vi "Pressure_Control.vi"() -> ()   [LabVIEW 2019]
uses:
  Pressure Control SubVIs/Device Data.ctl
  DevHandshake_elt.ctl
  <vilib>/Platform/TimedLoop/XDataNode/timing_clust.ctl
  <vilib>/Platform/TimedLoop/XDataNode/nitl_modes.ctl
  <vilib>/Platform/TimedLoop/XDataNode/wakeup.ctl
  octo-master/octo-master/DevHandshake.ctl
  <vilib>/platform/TimedLoop/XDataNode/XDataNode.xnode
  <vilib>/Platform/TimedLoop/XDataNode/XDNodeRunTimeDep.lvlib
panel:
  out "DevSave":T1
  out "Error Out":errorcluster
  in  "Current pressure status":string
  in  "Pressure tolerance %":sgl
  out "Status":string="NOT SYNC'D"
  out "Dev ID":string="pressureControl"
  in  "DevNum":i16=5
  out "Warning":bool
  out "Device Data":T2={"COM"=4, "Baud"=19200, "IDH"=0, "IDM"=0, "IDL"=0, "IDS"=0} {"IDS" format="%.0x"; "IDL" format="%.0x"; "IDM" format="%.0x"; "IDH" format="%.0x"}
  in  "SetPoint":sgl format="%.2f"
  in  "Write setpoint":bool
  in  "Read current setpoint":bool
  out "Unit":string
  out "Set Point Value":sgl format="%.2f"
  out "SetPoint %":sgl format="%.2f"
  in  "Lock to Network":bool
  out "Pressure Unit":string
  out "Pressure":sgl format="%.2f"
  in  "Read current pressure":bool
  in  "Message":string
  out "Function Output Comment":string
  in  "Start device":bool
  in  "Stop Button":bool
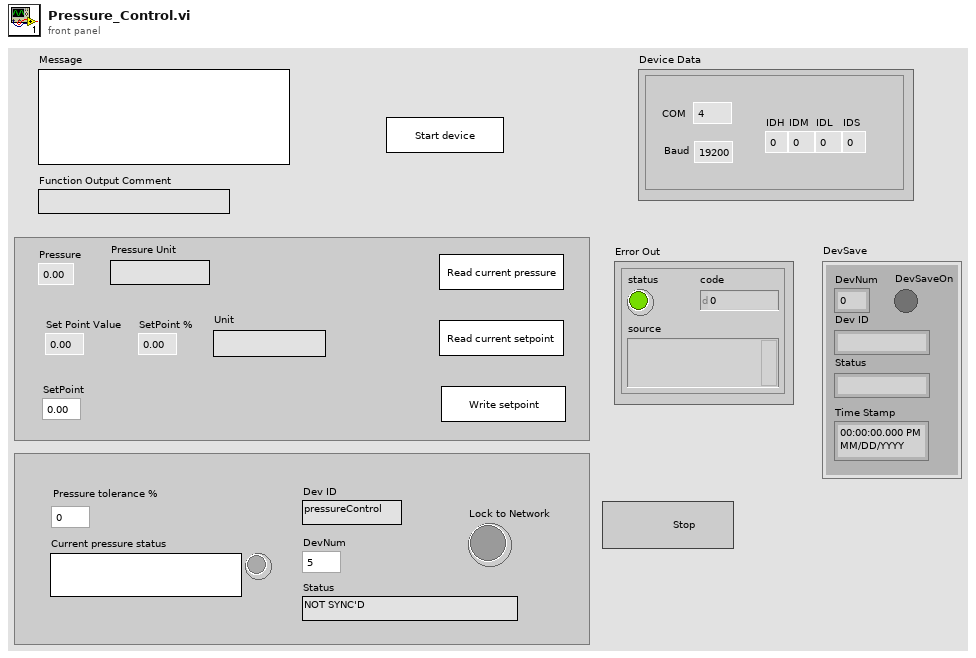
[diagram p1: front panel]
types:
  T1 = typedef "DevHandshake_elt.ctl" = cluster{"DevSaveOn":bool, "DevNum":i16, "Dev ID":string, "Status":string, "Time Stamp":timestamp}
  T2 = typedef "Device Data.ctl" = cluster{"COM":i32, "Baud":i32, "IDH":u8, "IDM":u8, "IDL":u8, "IDS":u8}
  T3 = typedef "XDNodeRunTimeDep.lvlib/timing_clust.ctl" = cluster{"Expected End [f-1]":u64, "Actual End [f-1]":u64, "Finished Late? [f-1]":bool, "Expected End [i-1]":u64, "Actual End [i-1]":u64, "Finished Late? [i-1]":bool, "Expected Start [i]":u64, "Actual Start [i]":u64, "Expected Start [f]":u64, "Actual Start [f]":u64, "Source Name":string, "Structure Name":string, "Period":i64, "Deadline":i64, "Offset":i64, "Start":i64, "Priority":i32, "Timeout":i32, "Mode":T4, "Wakeup Reason":T5, "Error":errorcluster, "Source Type":string, "Secondary Source Type":string, "Global End Time":u64, "Global Start Time":u64, "Frame Duration":u64, "Iteration Duration":u64, "Assigned CPU":i32, "I/O Scan Engine Mode":u32}
  T4 = typedef "XDNodeRunTimeDep.lvlib/nitl_modes.ctl" = enum32{"No Change", "Process missed periods, maintain original phase", "Discard missed periods, maintain original phase", "Process missed periods, ignore original phase", "Discard missed periods, ignore original phase"}
  T5 = typedef "XDNodeRunTimeDep.lvlib/wakeup.ctl" = enum32{"Normal", "Aborted", "Asynchronous wakeup", "Timing source error", "Timed loop error", "Timeout"}
  T6 = typedef "DevHandshake.ctl" = cluster{"DevSaveOn":bool, "DevNum":i16, "Dev ID":string, "Status":string, "Time Stamp":timestamp}[]
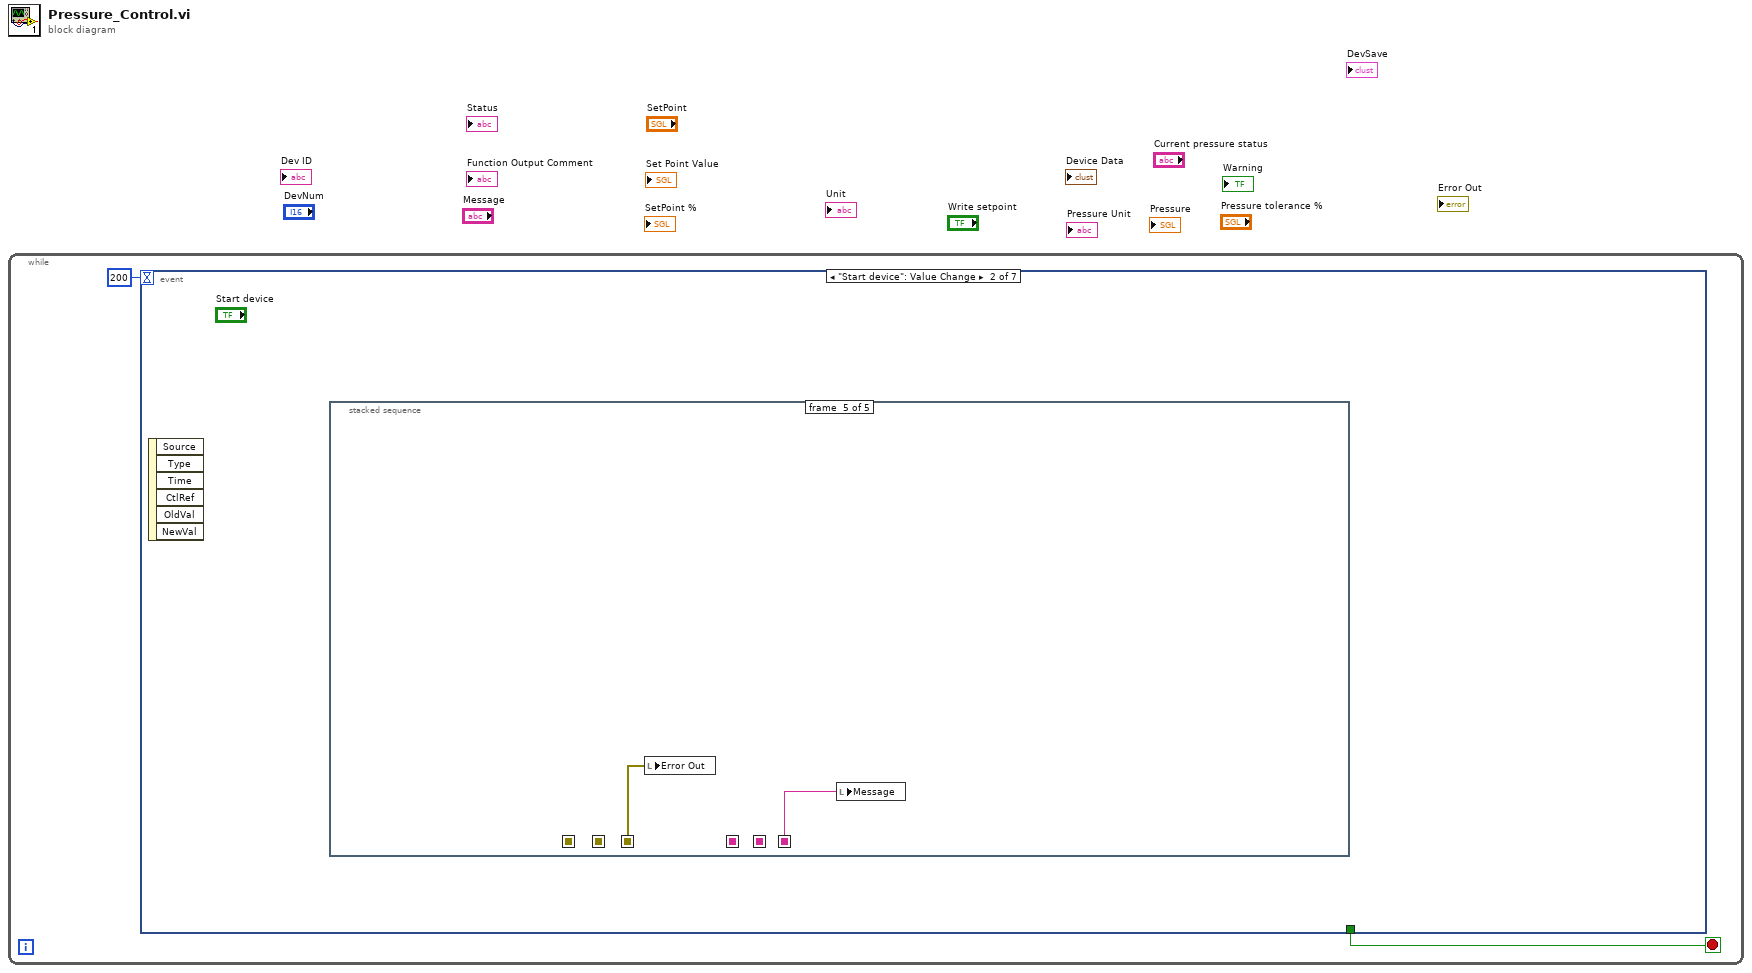
[diagram p0: block diagram]
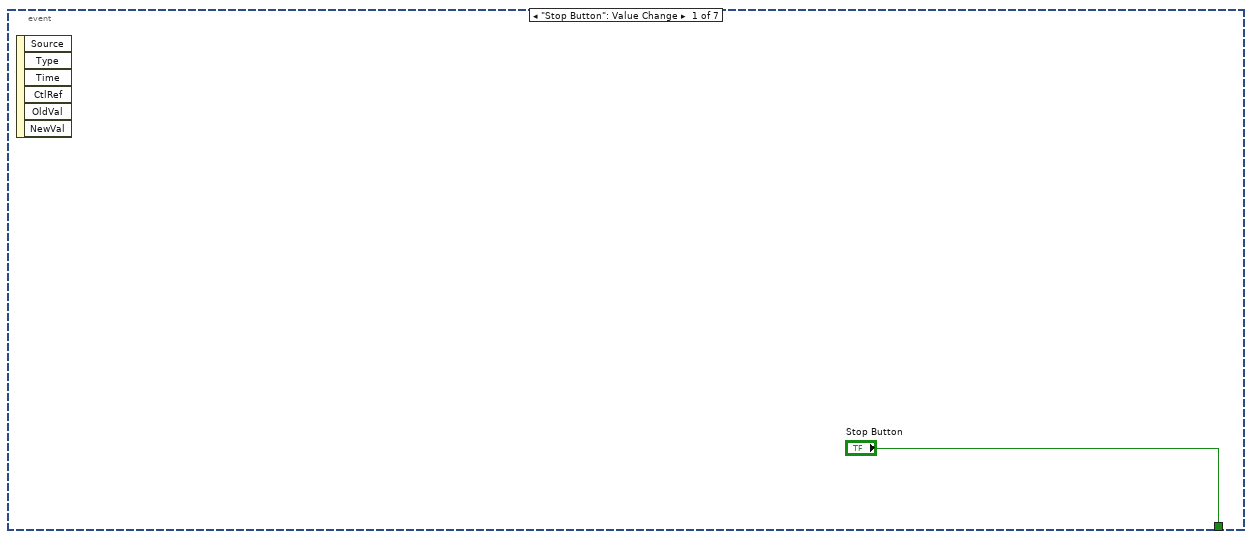
[diagram p2: hidden frame]
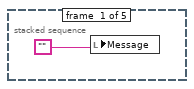
[diagram p3: hidden frame]
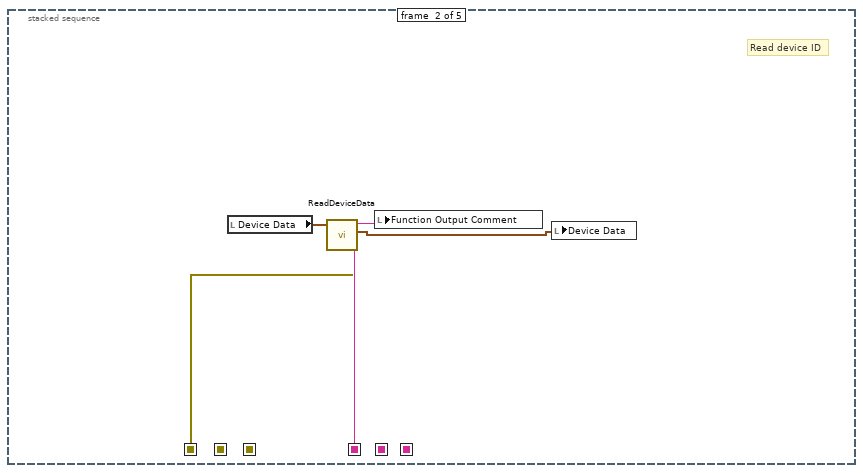
[diagram p4: hidden frame]
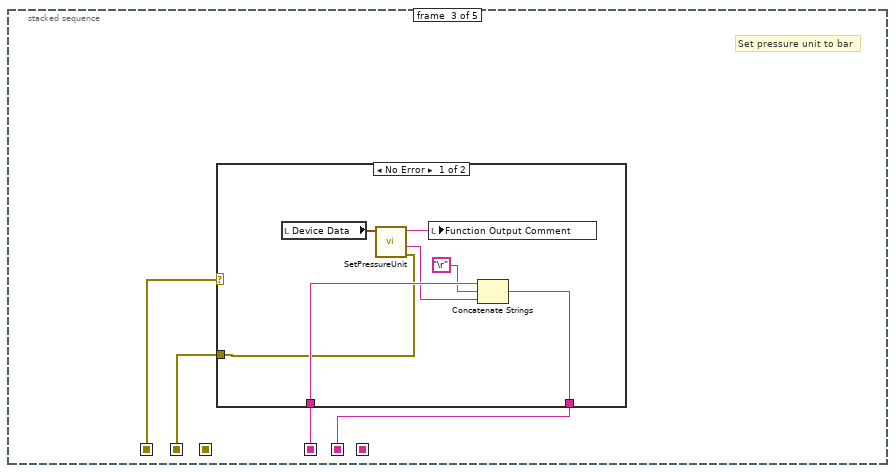
[diagram p5: hidden frame]
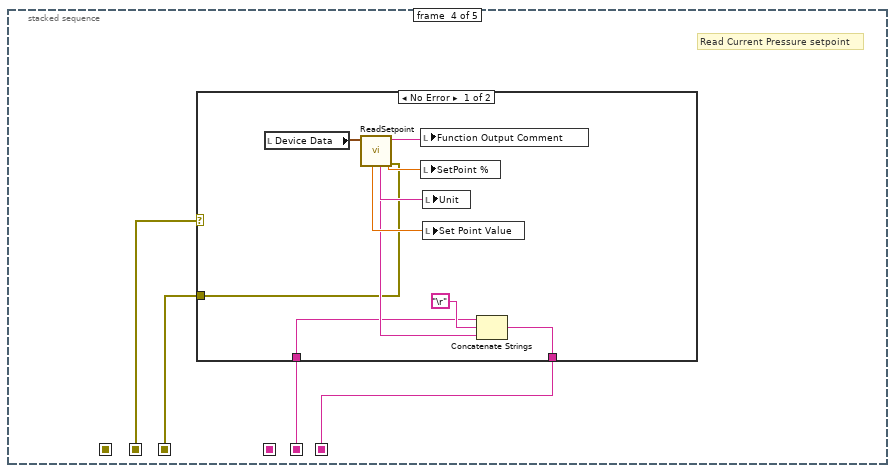
[diagram p7: hidden frame]
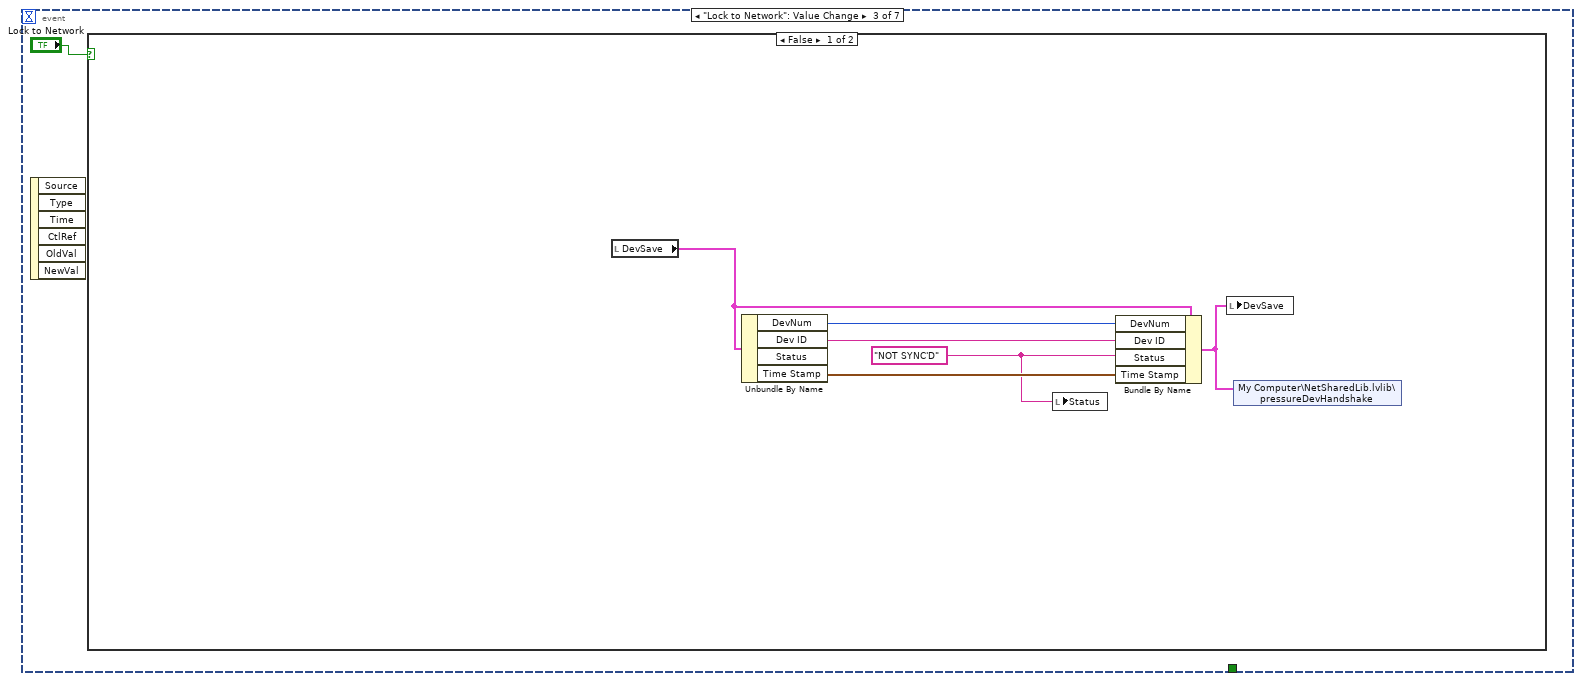
[diagram p9: hidden frame]
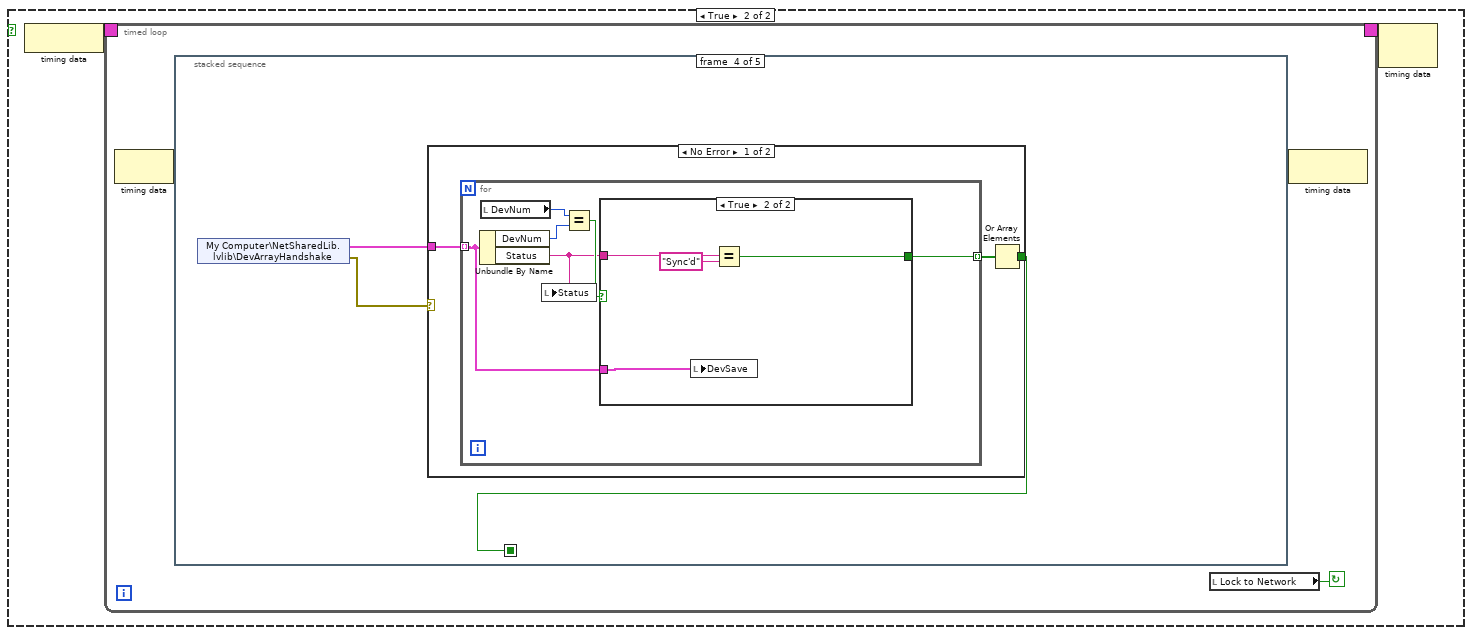
[diagram p10: hidden frame]
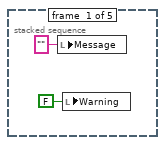
[diagram p11: hidden frame]
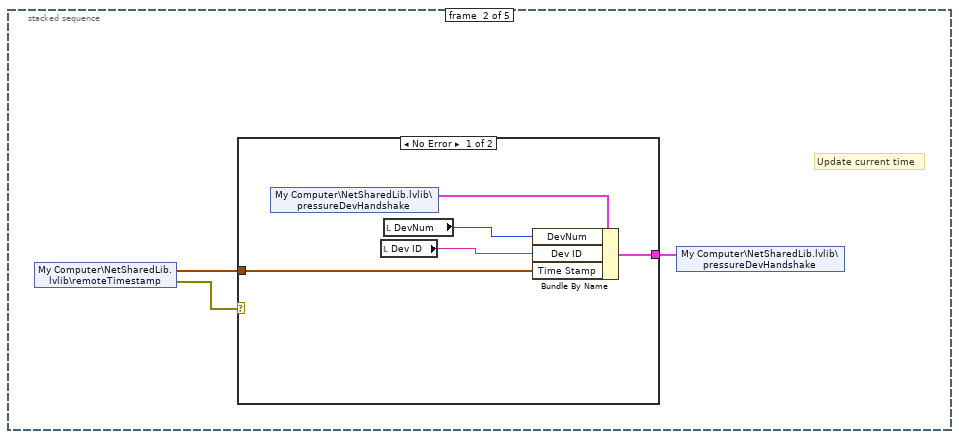
[diagram p12: hidden frame]
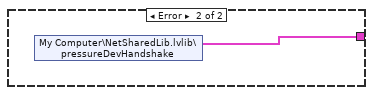
[diagram p13: hidden frame]
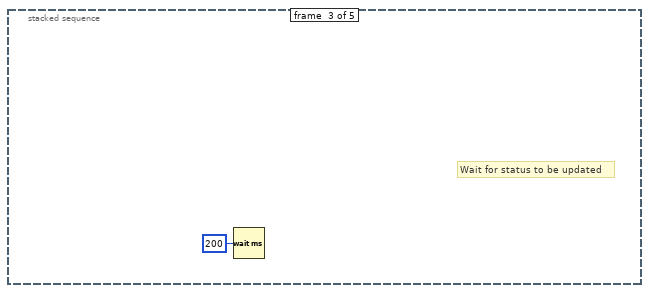
[diagram p14: hidden frame]
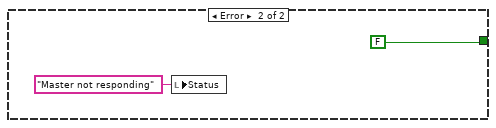
[diagram p16: hidden frame]
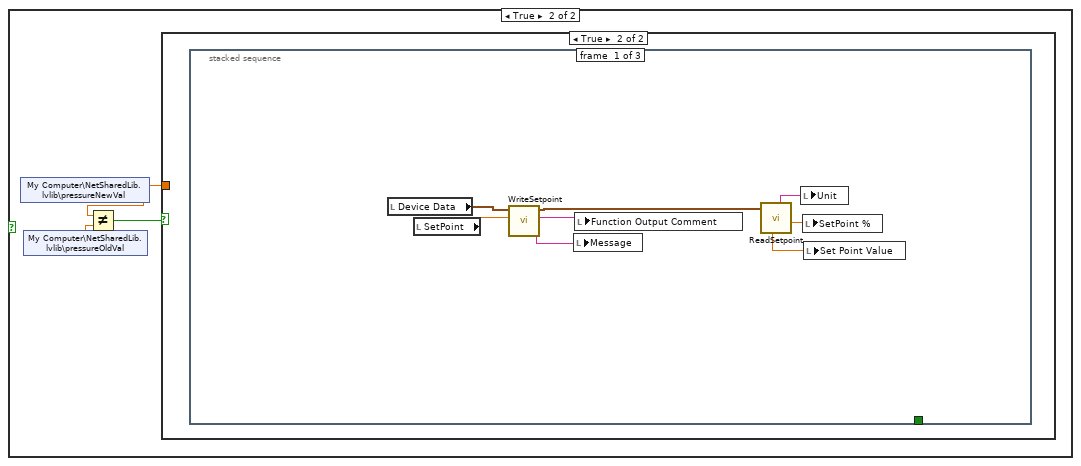
[diagram p18: hidden frame]
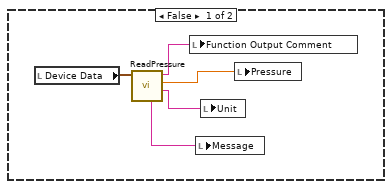
[diagram p19: hidden frame]
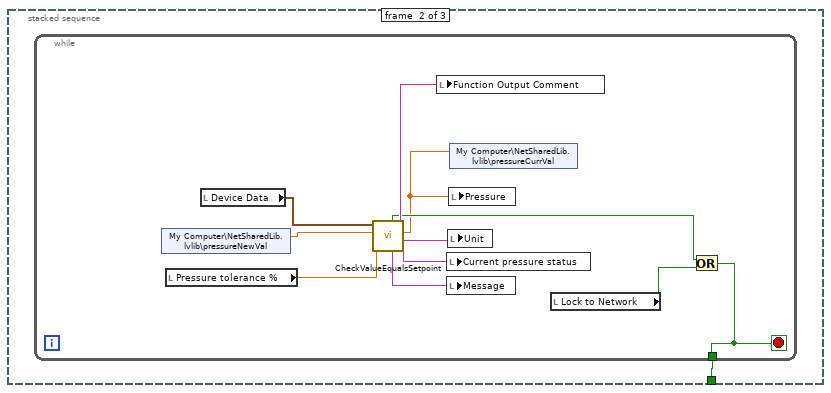
[diagram p20: hidden frame]
diagram:
  n1 = while {
    stop <- w2 stop-if-true
    n2 = event shown="[1] \"Start device\": Value Change" {
      selector: _ -> [_ _ _ _ _ _ _]
      dyn-events: _ -> [_ _ _ _ _ _ _]
      timeout: 200 -> [_ _ _ _ _ _ _]
      tunnel: ["Stop Button" _ _ _ _ _ _] -> w2
      event "Stop Button": Value Change {
        n3 = event-data() -> ()  [unwired: 1 in, 6 out]
      }
      event "Start device": Value Change {
        n4 = event-data() -> ()  [unwired: 1 in, 6 out]
        n5 = stacked-sequence {
          seq-local: [_ w8 _ _ _] -> [_ _ w13 _ _]
          seq-local: [_ _ w12 _ _] -> [_ _ _ w26 _]
          seq-local: [_ _ _ w25 _] -> [_ _ _ _ w40]
          seq-local: [_ w5 _ _ _] -> [_ _ w11 _ _]
          seq-local: [_ _ w10 _ _] -> [_ _ _ w24 _]
          seq-local: [_ _ _ w23 _] -> [_ _ _ _ w39]
          frame #0 {
            n6 = local write "Message"("") -> ()
          }
          frame #1 {
            # "Read device ID"
            n7 = local read "Device Data"() -> (w6:T2)
            n8 = call "ReadDeviceData.vi"("Device Data in"=w6) -> ("Error Out"=w5:errorcluster, "Message"=w8:string, "Device Data out"=w7:T2, "Function Output Comment"=w9:string)  [unwired: 7 in]
            n9 = local write "Function Output Comment"(w9) -> ()
            n10 = local write "Device Data"(w7) -> ()
          }
          frame #2 {
            # "Set pressure unit to bar"
            n11 = case shown="No Error" w11 {
              selector: w11 -> [_ w21]
              tunnel: w13 -> [w18 w22]
              tunnel: [w15 w22] -> w12
              tunnel: [w14 w21] -> w10
              frame No Error {
                n12 = local read "Device Data"() -> (w19:T2)
                n13 = call "SetPressureUnit.vi"("Device Data in"=w19) -> ("Error Out"=w14:errorcluster, "Message"=w17:string, "Function Output Comment"=w20:string)  [unwired: 7 in, 1 out]
                n14 = local write "Function Output Comment"(w20) -> ()
                n15 = Concatenate Strings(w18, "\r", w17) -> (w15:string)
              }
              frame Error {
              }
            }
          }
          frame #3 {
            # "Read Current Pressure setpoint"
            n16 = case shown="No Error" w24 {
              selector: w24 -> [_ w38]
              tunnel: w26 -> [w29 w37]
              tunnel: [w28 w37] -> w25
              tunnel: [w27 w38] -> w23
              frame No Error {
                n17 = local read "Device Data"() -> (w32:T2)
                n18 = call "ReadSetpoint.vi"("Device Data in"=w32) -> ("Error Out"=w27:errorcluster, "SetPoint %"=w35:sgl, "Function Output Comment"=w36:string, "Unit"=w33:string, "Message"=w30:string, "SetPointValue"=w34:sgl)  [unwired: 4 in, 1 out]
                n19 = local write "Function Output Comment"(w36) -> ()
                n20 = local write "SetPoint %"(w35) -> ()
                n21 = local write "Unit"(w33) -> ()
                n22 = local write "Set Point Value"(w34) -> ()
                n23 = Concatenate Strings(w29, "\r", w30) -> (w28:string)
              }
              frame Error {
              }
            }
          }
          frame #4 {
            n24 = local write "Error Out"(w39) -> ()
            n25 = local write "Message"(w40) -> ()
          }
        }
      }
      event "Lock to Network": Value Change {
        n26 = event-data() -> ()  [unwired: 1 in, 6 out]
        n27 = case shown="False" "Lock to Network" {
          frame False {
            w42 = "NOT SYNC'D"
            n28 = local read "DevSave"() -> (w43:T1)
            n29 = Unbundle By Name(w43) -> ("DevNum"=w47:i16, "Dev ID"=w46:string, "Time Stamp"=w45:timestamp)  [unwired: 1 out]
            n30 = local write "Status"(w42) -> ()
            n31 = Bundle By Name(cluster=w43, "DevNum"=w47, "Dev ID"=w46, "Status"=w42, "Time Stamp"=w45) -> (w44:T1)
            n32 = local write "DevSave"(w44) -> ()
            n33 = shared-variable "My Computer\\NetSharedLib.lvlib\\pressureDevHandshake"(w44) -> ()  [unwired: 1 in, 1 out]
          }
          frame True {
            n34 = node-c288() -> (w49:T3)
            n35 = timed-loop {
              timing: w49 -> [_]
              timing-out: [_] -> w48
              stop <- w50 continue-if-true
              n36 = node-c288() -> ()  [unwired: 1 in, 1 out]
              n37 = stacked-sequence {
                seq-local: [_ _ _ w66 _] -> [_ _ _ _ w84]
                frame #0 {
                  n38 = local write "Message"("" ("Message")) -> ()
                  n39 = local write "Warning"(FALSE ("Warning")) -> ()
                }
                frame #1 {
                  # "Update current time"
                  n40 = shared-variable "My Computer\\NetSharedLib.lvlib\\remoteTimestamp"() -> (w57:timestamp, error out=w55:errorcluster)  [unwired: 1 in]
                  n41 = case shown="No Error" w55 {
                    tunnel: w57 -> [w60 _]
                    tunnel: [w58 w63] -> w56
                    frame No Error {
                      n42 = shared-variable "My Computer\\NetSharedLib.lvlib\\pressureDevHandshake"() -> (w59:T1)  [unwired: 1 in, 1 out]
                      n43 = local read "Dev ID"() -> (w62:string)
                      n44 = local read "DevNum"() -> (w61:i16)
                      n45 = Bundle By Name(cluster=w59, "DevNum"=w61, "Dev ID"=w62, "Time Stamp"=w60) -> (w58:T1)
                    }
                    frame Error {
                      n46 = shared-variable "My Computer\\NetSharedLib.lvlib\\pressureDevHandshake"() -> (w63:T1)  [unwired: 1 in, 1 out]
                    }
                  }
                  n47 = shared-variable "My Computer\\NetSharedLib.lvlib\\pressureDevHandshake"(w56) -> ()  [unwired: 1 in, 1 out]
                }
                frame #2 {
                  # "Wait for status to be updated"
                  n48 = Wait (ms)(milliseconds to wait=u32 200) -> ()  [unwired: 1 out]
                }
                frame #3 {
                  n49 = shared-variable "My Computer\\NetSharedLib.lvlib\\DevArrayHandshake"() -> (w67:T6, error out=w65:errorcluster)  [unwired: 1 in]
                  n50 = case shown="No Error" w65 {
                    tunnel: w67 -> [w70 _]
                    tunnel: [w68 FALSE] -> w66
                    frame No Error {
                      n51 = for {
                        tunnel: w70 -> [w71] mode=indexing
                        tunnel: [w73] -> w69 mode=indexing
                        n52 = Unbundle By Name(w71) -> ("DevNum"=w76:i16, "Status"=w72:string)
                        n53 = local read "DevNum"() -> (w75:i16)
                        n54 = local write "Status"(w72) -> ()
                        n55 = Equal?(x=w75, y=w76) -> (x = y?=w74:bool)
                        n56 = case shown="True" w74 {
                          selector: w74 -> [w77 _]
                          tunnel: w72 -> [_ w81]
                          tunnel: [w77 w79] -> w73
                          tunnel: w71 -> [_ w78]
                          frame False {
                          }
                          frame True {
                            n57 = local write "DevSave"(w78) -> ()
                            n58 = Equal?(x=w81, y="Sync'd") -> (x = y?=w79:bool)
                          }
                        }
                      }
                      n59 = Or Array Elements(Boolean array=w69) -> (logical OR=w68:bool)
                    }
                    frame Error {
                      n60 = local write "Status"("Master not responding" ("Status")) -> ()
                    }
                  }
                }
                frame #4 {
                  n61 = case shown="False" w84 {
                    frame False {
                    }
                    frame True {
                      n62 = shared-variable "My Computer\\NetSharedLib.lvlib\\pressureNewVal"() -> (w85:sgl)  [unwired: 1 in, 1 out]
                      n63 = shared-variable "My Computer\\NetSharedLib.lvlib\\pressureOldVal"() -> (w87:sgl)  [unwired: 1 in, 1 out]
                      n64 = Not Equal?(x=w85, y=w87) -> (x != y?=w86:bool)
                      n65 = case shown="True" w86 {
                        tunnel: w85 -> [_ _]
                        frame False {
                          n66 = local read "Device Data"() -> (w92:T2)
                          n67 = call "ReadPressure.vi"("Device Data"=w92) -> ("Unit"=w88:string, "Pressure"=w90:sgl, "Function Output Comment"=w91:string, "Message"=w89:string)  [unwired: 7 in]
                          n68 = local write "Function Output Comment"(w91) -> ()
                          n69 = local write "Message"(w89) -> ()
                          n70 = local write "Unit"(w88) -> ()
                          n71 = local write "Pressure"(w90) -> ()
                        }
                        frame True {
                          n72 = stacked-sequence {
                            tunnel: [_ w101 _] -> _
                            frame #0 {
                              n73 = local read "Device Data"() -> (w96:T2)
                              n74 = local read "SetPoint"() -> (w98:sgl)
                              n75 = call "WriteSetpoint.vi"("SetPoint"=w98, "Device Data"=w96) -> ("Message"=w97:string, "Function Output Comment"=w99:string, "Device Data OUT"=w100:T2)  [unwired: 6 in]
                              n76 = local write "Message"(w97) -> ()
                              n77 = local write "Function Output Comment"(w99) -> ()
                              n78 = call "ReadSetpoint.vi"("Device Data in"=w100) -> ("SetPoint %"=w95:sgl, "Unit"=w93:string, "SetPointValue"=w94:sgl)  [unwired: 4 in, 4 out]
                              n79 = local write "Unit"(w93) -> ()
                              n80 = local write "SetPoint %"(w95) -> ()
                              n81 = local write "Set Point Value"(w94) -> ()
                            }
                            frame #1 {
                              n82 = while {
                                tunnel: [w104] -> w101
                                stop <- w104 stop-if-true
                                n83 = shared-variable "My Computer\\NetSharedLib.lvlib\\pressureNewVal"() -> (w107:sgl)  [unwired: 1 in, 1 out]
                                n84 = local read "Pressure tolerance %"() -> (w108:sgl)
                                n85 = local read "Device Data"() -> (w112:T2)
                                n86 = call "CheckValueEqualsSetpoint.vi"("Pressure tolerance %"=w108, "PressureNewVal"=w107, "Device Data"=w112) -> ("Current pressure status"=w106:string, "Unit"=w109:string, "Pressure"=w102:sgl, "Function Output Comment"=w111:string, "Message"=w110:string, "PeqPSet ?"=w105:bool)  [unwired: 3 in]
                                n87 = local write "Function Output Comment"(w111) -> ()
                                n88 = local write "Current pressure status"(w106) -> ()
                                n89 = local write "Message"(w110) -> ()
                                n90 = local write "Unit"(w109) -> ()
                                n91 = local write "Pressure"(w102) -> ()
                                n92 = shared-variable "My Computer\\NetSharedLib.lvlib\\pressureCurrVal"(w102) -> ()  [unwired: 1 in, 1 out]
                                n93 = local read "Lock to Network"() -> (w103:bool)
                                n94 = Or(x=w105, y=w103) -> (x .or. y?=w104:bool)
                              }
                            }
                            frame #2 {
                              n95 = local read "Lock to Network"() -> (w113:bool)
                              n96 = case shown="True" w113 {
                                frame False {
                                n97 = local read "Current pressure status"() -> (w117:string)
                                n98 = Concatenate Strings(w117, "\r" ("string"), "Connection to network was unlocked by user  " ("string")) -> (w114:string)
                                n99 = local write "Current pressure status"(w114) -> ()
                                }
                                frame True {
                                n100 = shared-variable "My Computer\\NetSharedLib.lvlib\\pressureNewVal"() -> (w118:sgl)  [unwired: 1 in, 1 out]
                                n101 = shared-variable "My Computer\\NetSharedLib.lvlib\\pressureOldVal"(w118) -> ()  [unwired: 1 in, 1 out]
                                }
                              }
                            }
                          }
                        }
                      }
                    }
                  }
                }
              }
              n102 = local read "Lock to Network"() -> (w50:bool)
              n103 = node-c288() -> ()  [unwired: 1 in, 1 out]
            }
            n104 = node-c288(w48) -> ()  [unwired: 1 out]
          }
        }
      }
      event "Read current pressure": Value Change {
        n105 = event-data() -> ()  [unwired: 1 in, 6 out]
        n106 = local read "Device Data"() -> (w122:T2)
        n107 = call "ReadPressure.vi"("Device Data"=w122) -> ("Unit"=w123:string, "Pressure"=w121:sgl, "Function Output Comment"=w125:string, "Message"=w124:string)  [unwired: 7 in]
        n108 = local write "Pressure Unit"(w123) -> ()
        n109 = local write "Message"(w124) -> ()
        n110 = local write "Function Output Comment"(w125) -> ()
        n111 = shared-variable "My Computer\\NetSharedLib.lvlib\\pressureCurrVal"(w121) -> ()  [unwired: 1 in, 1 out]
        n112 = local write "Pressure"(w121) -> ()
      }
      event "Read current setpoint": Value Change {
        n113 = event-data() -> ()  [unwired: 1 in, 6 out]
        n114 = local read "Device Data"() -> (w131:T2)
        n115 = call "ReadSetpoint.vi"("Device Data in"=w131) -> ("SetPoint %"=w129:sgl, "Function Output Comment"=w126:string, "Unit"=w130:string, "Message"=w127:string, "SetPointValue"=w128:sgl)  [unwired: 4 in, 2 out]
        n116 = local write "Message"(w127) -> ()
        n117 = local write "Unit"(w130) -> ()
        n118 = local write "Set Point Value"(w128) -> ()
        n119 = local write "Function Output Comment"(w126) -> ()
        n120 = local write "SetPoint %"(w129) -> ()
      }
      event "Write setpoint": Value Change {
        n121 = event-data() -> ()  [unwired: 1 in, 6 out]
        n122 = stacked-sequence {
          frame #0 {
            n123 = local read "Device Data"() -> (w132:T2)
            n124 = local read "SetPoint"() -> (w134:sgl)
            n125 = call "WriteSetpoint.vi"("SetPoint"=w134, "Device Data"=w132) -> ("Message"=w133:string, "Function Output Comment"=w135:string)  [unwired: 6 in, 1 out]
            n126 = local write "Function Output Comment"(w135) -> ()
            n127 = local write "Message"(w133) -> ()
          }
          frame #1 {
            n128 = local read "Device Data"() -> (w141:T2)
            n129 = call "ReadSetpoint.vi"("Device Data in"=w141) -> ("SetPoint %"=w140:sgl, "Function Output Comment"=w136:string, "Unit"=w138:string, "Message"=w137:string, "SetPointValue"=w139:sgl)  [unwired: 4 in, 2 out]
            n130 = local write "SetPoint %"(w140) -> ()
            n131 = local write "Set Point Value"(w139) -> ()
            n132 = local write "Function Output Comment"(w136) -> ()
            n133 = local write "Message"(w137) -> ()
            n134 = local write "Unit"(w138) -> ()
          }
        }
      }
      event Timeout {
        n135 = event-data() -> ()  [unwired: 1 in, 3 out]
        n136 = local read "Device Data"() -> (w143:T2)
        n137 = call "ReadPressure.vi"("Device Data"=w143) -> ("Unit"=w144:string, "Pressure"=w142:sgl, "Function Output Comment"=w146:string, "Message"=w145:string)  [unwired: 7 in]
        n138 = local write "Function Output Comment"(w146) -> ()
        n139 = local write "Pressure Unit"(w144) -> ()
        n140 = local write "Message"(w145) -> ()
        n141 = shared-variable "My Computer\\NetSharedLib.lvlib\\pressureCurrVal"(w142) -> ()  [unwired: 1 in, 1 out]
        n142 = local write "Pressure"(w142) -> ()
      }
    }
  }
